vi "Find Expression in Array of Strings.vi"(3 "Expression to find":string, 4 "String Array":string[](array[string])) -> (0 "Array Indexes":i32[](array[numeric]), 1 "Matching Strings":string[](array[string]))   [LabVIEW 2016, in "WSsupport.lvlib"]
uses:
  WSsupport.lvlib
  <vilib>/regexp/Match Regular Expression.xnode
panel:
  out "error out":errorcluster
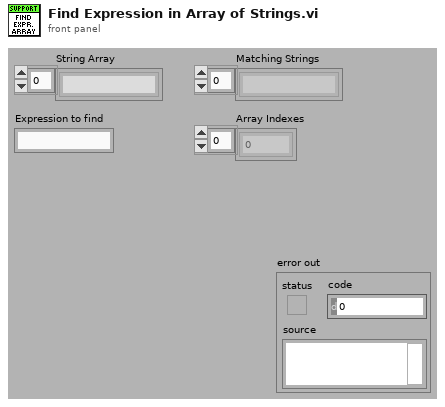
[diagram p1: front panel]
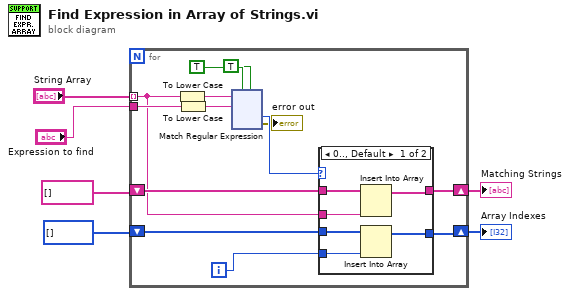
[diagram p0: block diagram]
diagram:
  n1 = for {
    tunnel: "String Array" -> [w13] mode=indexing
    shift-right: [w17] -> w4
    shift-left: string[] [] -> [w18]
    tunnel: "Expression to find" -> [w19]
    shift-right: [w15] -> w1
    shift-left: i32[] [] -> [w16]
    i -> [w14]
    n2 = To Lower Case(string=w13) -> (all lower case string=w8:string)
    n3 = To Lower Case(string=w19) -> (all lower case string=w7:string)
    n4 = xnode "Match Regular Expression"("input string"=w8, "regular expression"=w7, "ignore case? (F)"=TRUE, "multiline? (F)"=TRUE) -> ("offset past match"=w11:i32, "error out"=→"error out":errorcluster)  [unwired: 2 in, 3 out]
    n5 = case shown="0.., Default" w11 {
      tunnel: w18 -> [w136 w138]
      tunnel: [w134 w138] -> w17
      tunnel: w13 -> [w135 _]
      tunnel: w16 -> [w133 w137]
      tunnel: [w132 w137] -> w15
      tunnel: w14 -> [w131 _]
      frame 0.., Default {
        n6 = Insert Into Array(array=w136, new element=w135) -> (w134:string[])  [unwired: 1 in]
        n7 = Insert Into Array(array=w133, new element=w131) -> (w132:i32[])  [unwired: 1 in]
      }
      frame -1 {
      }
    }
  }
  "Matching Strings" <- w4
  "Array Indexes" <- w1
